vi "Error Converter (ErrCode or Status).vi"(8 "error in (no error)":errorcluster caption="Fehler (Eingang, kein Fehler)", 11 "error code":i32 caption="Fehlercode") -> (0 "error out":errorcluster caption="Fehler (Ausgang)")   [LabVIEW 2021, in "labbCAN_DigIO_API.lvlib"]
uses:
  labbCAN_DigIO_API.lvlib
  labbCAN_Bus_API/labbCAN_Bus_API.lvlib
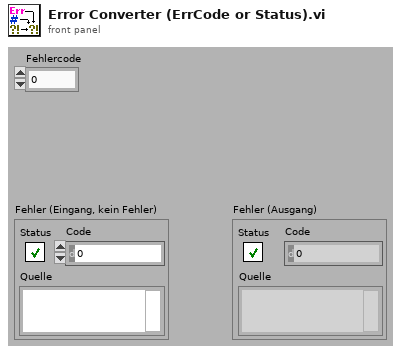
[diagram p1: front panel]
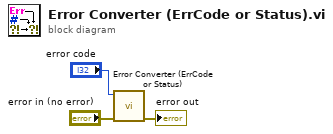
[diagram p0: block diagram]
diagram:
  n1 = call "Error Converter (ErrCode or Status).vi"("error in (no error)"="error in (no error)", "error code"="error code") -> ("error out"=→"error out":errorcluster)  [unwired: 9 in]
